vi "测试配置文件生成.vi"() -> ()   [LabVIEW 2013]
uses:
  <vilib>/Utility/config.llb/Write Key (String).vi
  <vilib>/Utility/config.llb/NI_LVConfig.lvlib
panel:
  in  "总电流":bool
  in  "外部总压":bool
  in  "内部总压":bool
  in  "选项卡控件":enum32{"关键配置", "功能测试"}(tab)
  in  "保存 2":bool
  in  "BMU合成程序全名-用于仿真器刷写":path
  in  "内部CAN波特率":enum16{"250K", "500K"}(ring)
  in  "整车CAN波特率":enum16{"250K", "500K"}(ring)
  in  "充电CAN波特率":enum16{"250K", "500K"}(ring)
  in  "BCU应用程序全名-用于在线更新程序":path
  in  "BMU个数":dbl
  in  "BMU应用程序全名 2":string[][](table)
  in  "BCU合成程序全名-用于仿真器刷写":path
  in  "配置文件全名":path
  in  "CP":bool
  in  "AI2":bool
  in  "AI1":bool
  in  "CC2":bool
  in  "CC":bool
  in  "全部忽略":bool
  in  "全部选择":bool
  in  "DO2":bool
  in  "DO1":bool
  in  "DI4":bool
  in  "DI3":bool
  in  "DI2":bool
  in  "DI1":bool
  in  "加热继电器":bool
  in  "风机继电器":bool
  in  "充电继电器":bool
  in  "预充继电器":bool
  in  "总负继电器":bool
  in  "总正继电器":bool
  in  "充电CAN":bool
  in  "整车CAN":bool
  in  "写入至从板号":dbl=1.0 min=1.0 max=30.0
  in  "更新至指定BMU号":bool
  in  "BMU应用程序全名":path
  in  "配置到全部BMU":bool
  out "取消":bool
  out "确定并启动":bool
  in  "自适就CAN卡类型":bool=TRUE
  in  "退出":bool
  in  "保存":bool
  in  "error in":errorcluster caption="错误输入"
  # "自动化测试配置文件生成器"
  # "将BMU应用程序全名："
  # "请勾选需要生产测试的功能........"
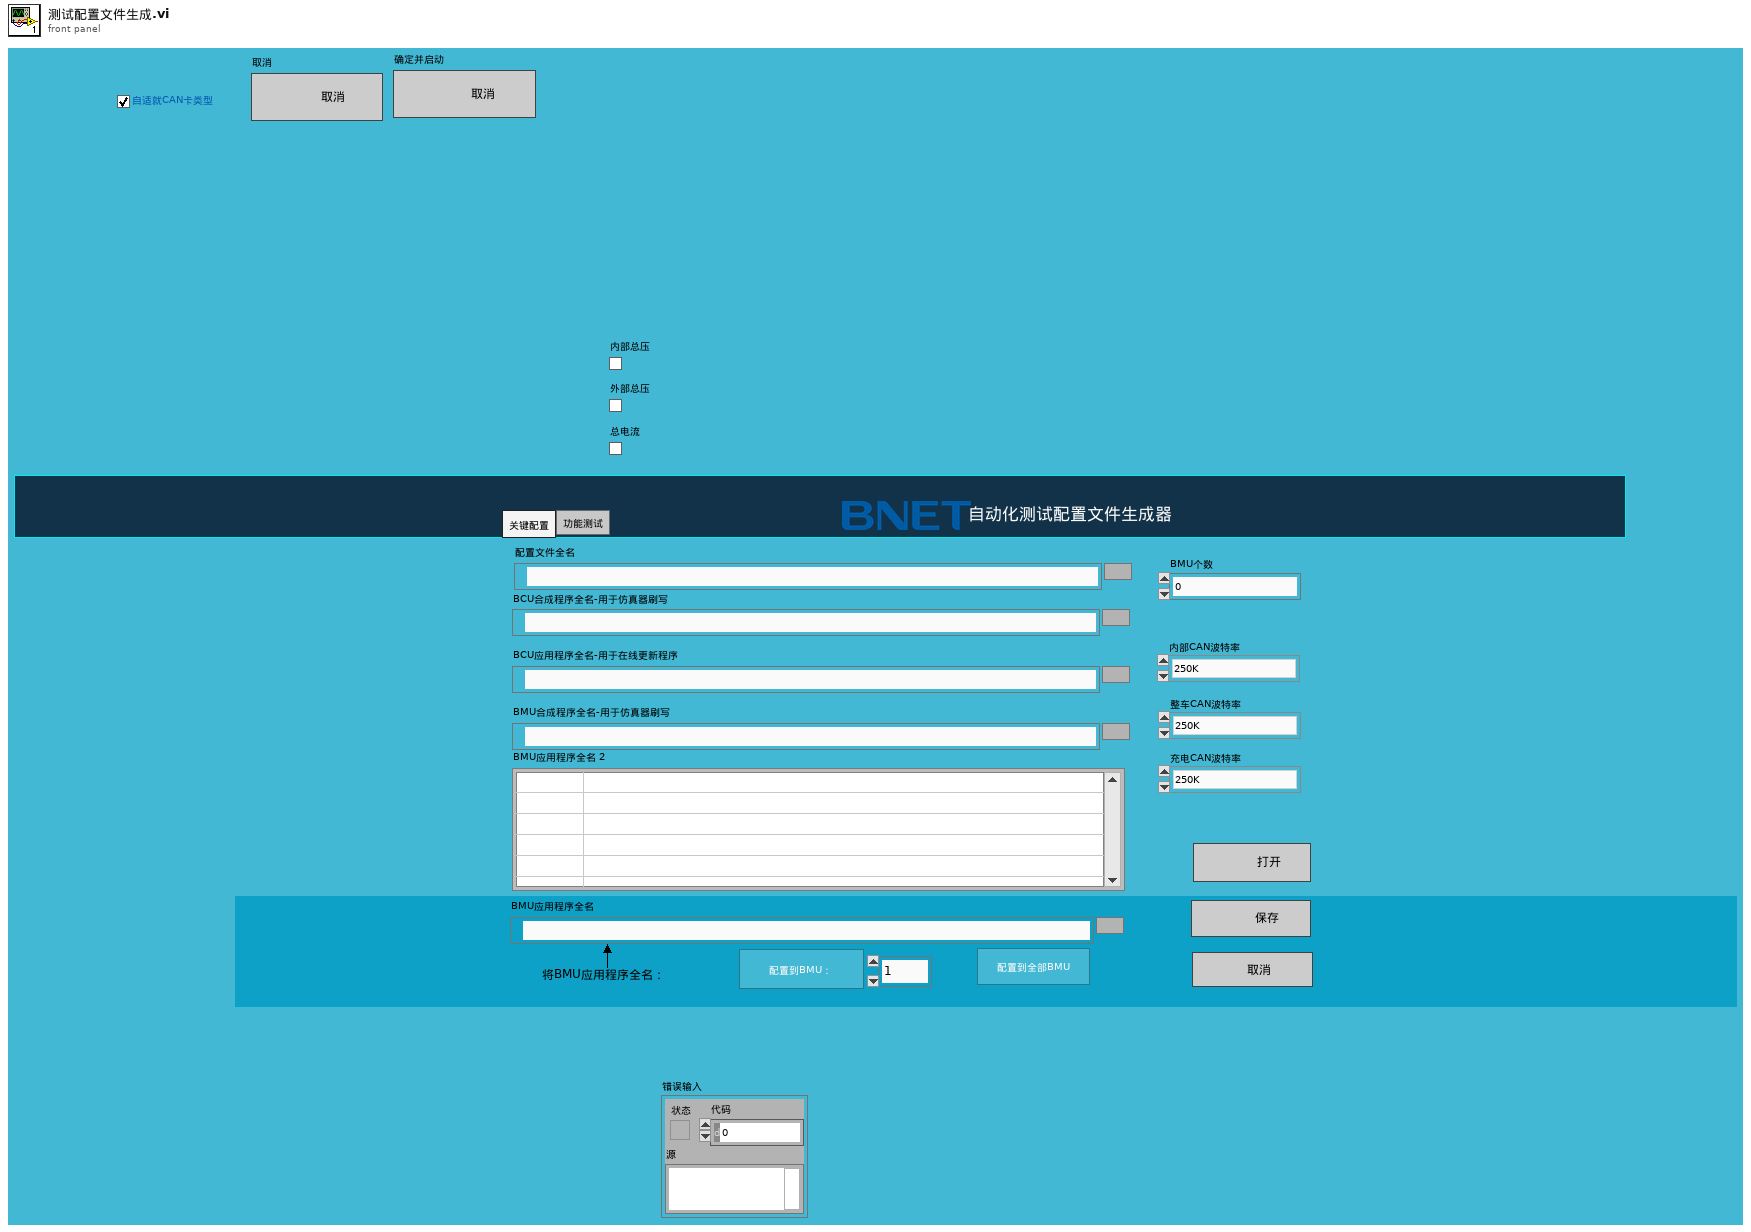
[diagram p1: front panel]
types:
  T1 = typedef "NI_LVConfig.lvlib/Config Data RefNum.ctl" = refnum<k1>
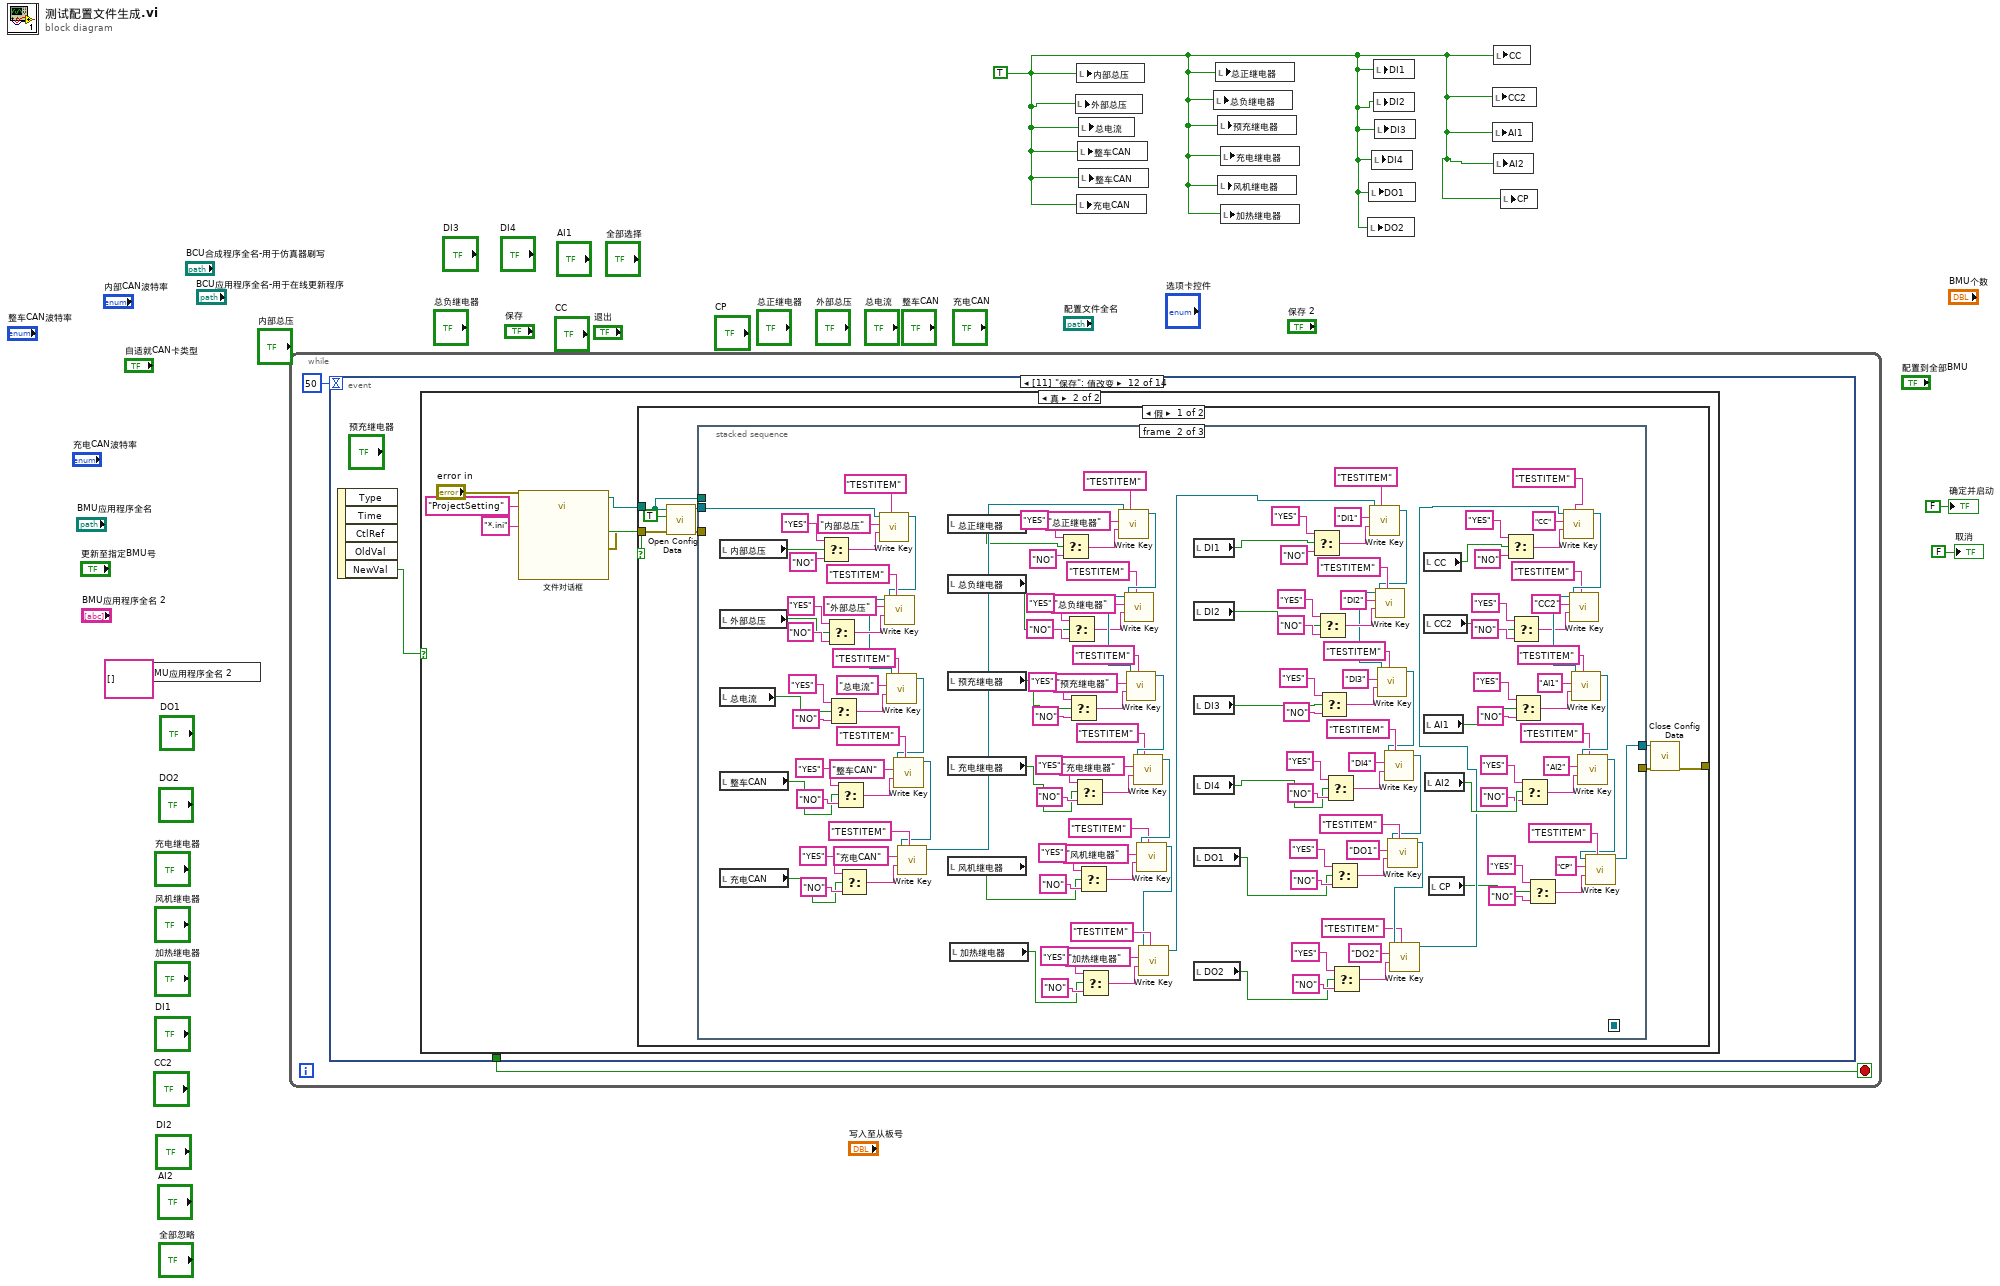
[diagram p0: block diagram]
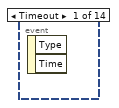
[diagram p2: hidden frame]
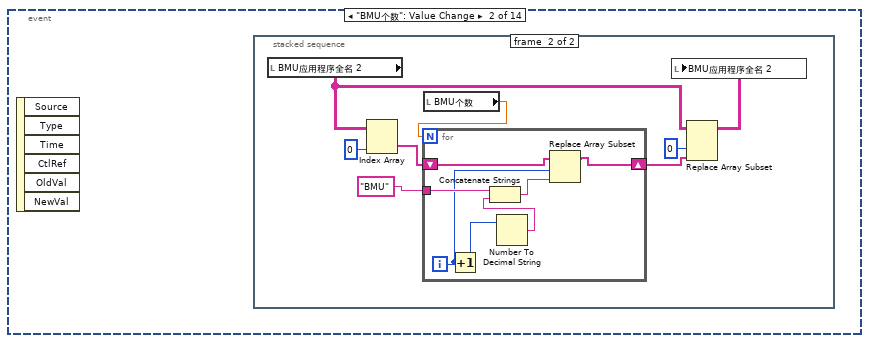
[diagram p3: hidden frame]
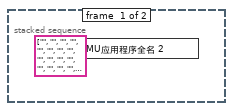
[diagram p4: hidden frame]
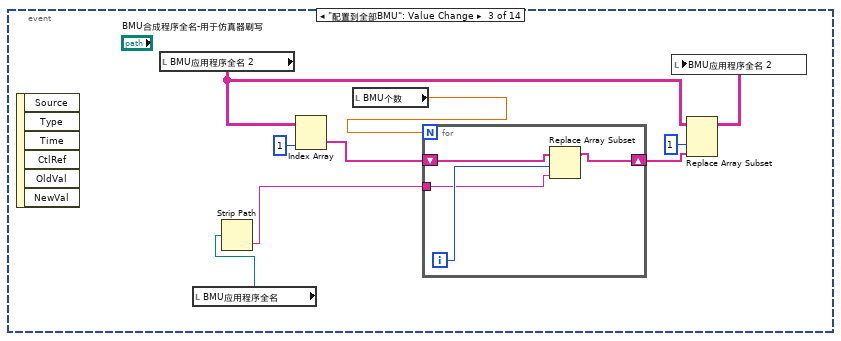
[diagram p5: hidden frame]
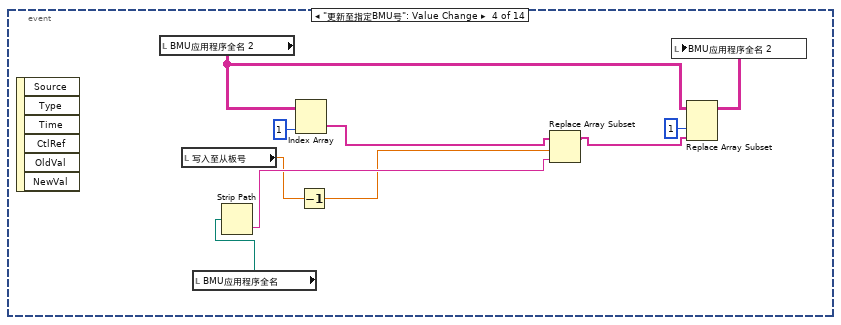
[diagram p6: hidden frame]
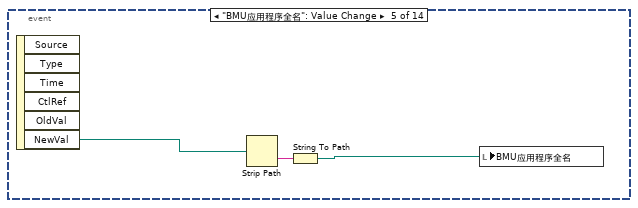
[diagram p7: hidden frame]
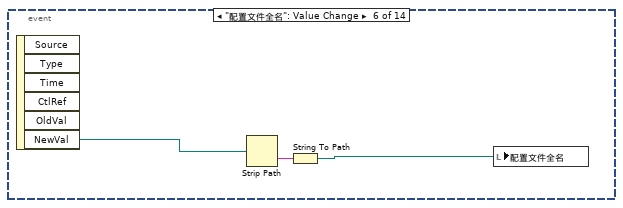
[diagram p8: hidden frame]
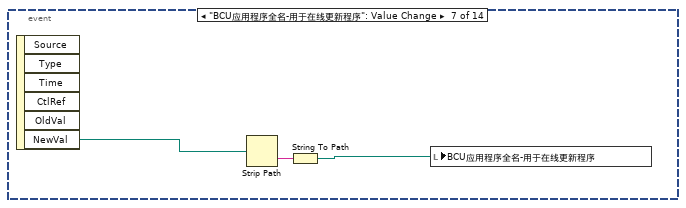
[diagram p9: hidden frame]
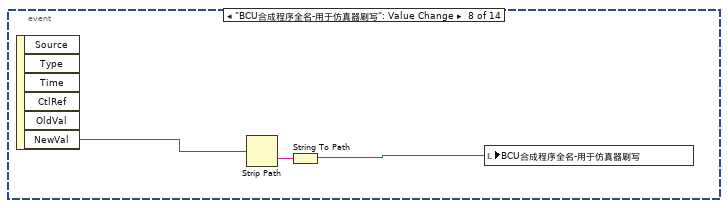
[diagram p10: hidden frame]
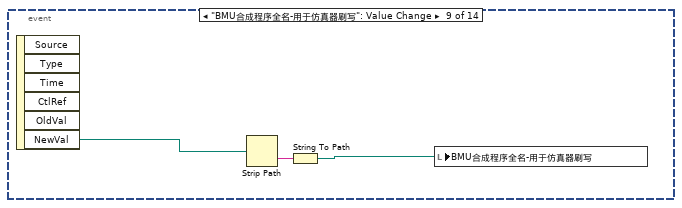
[diagram p11: hidden frame]
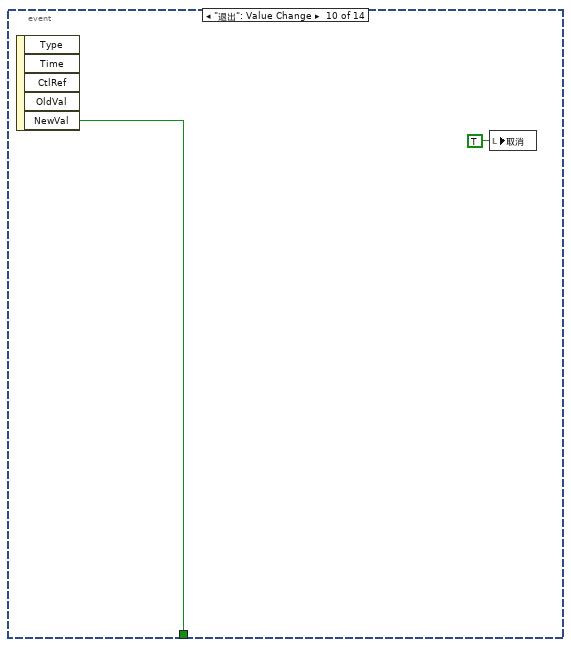
[diagram p12: hidden frame]
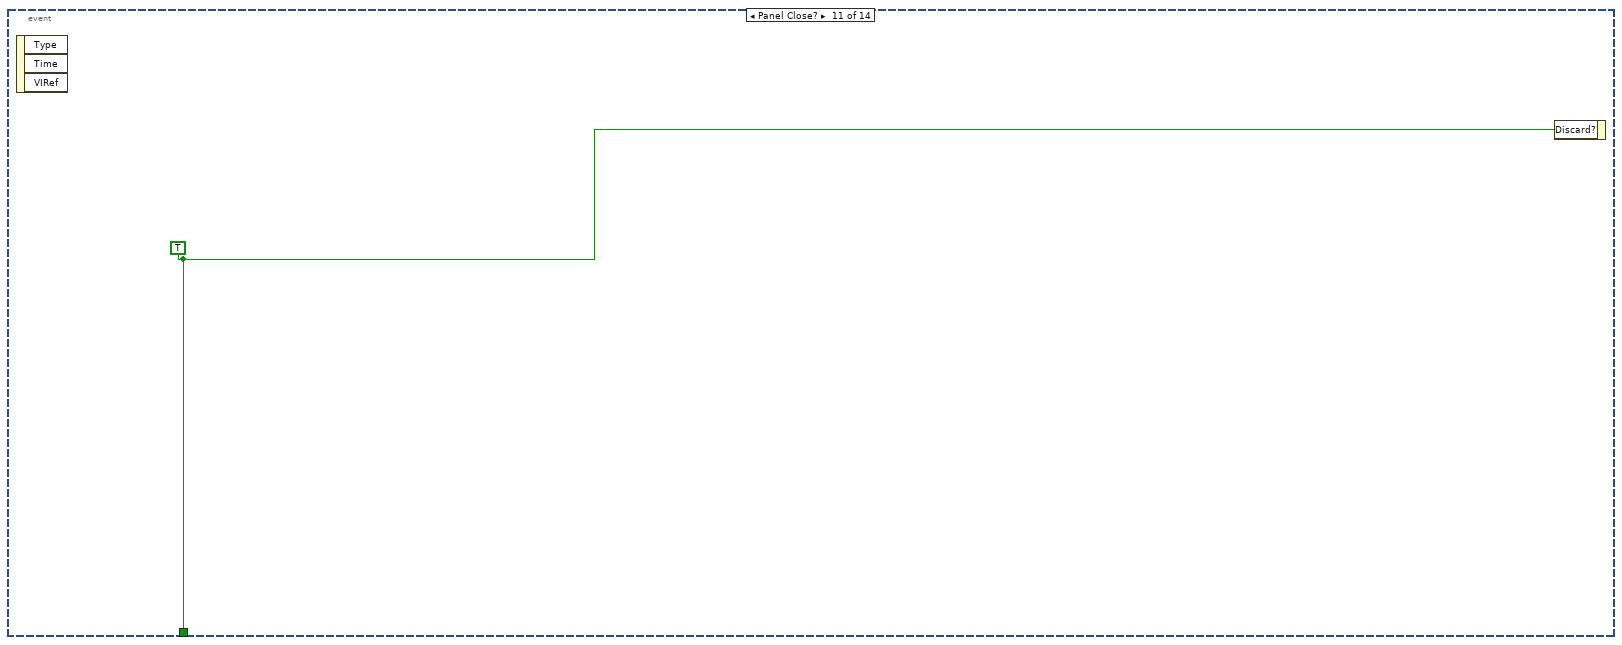
[diagram p13: hidden frame]
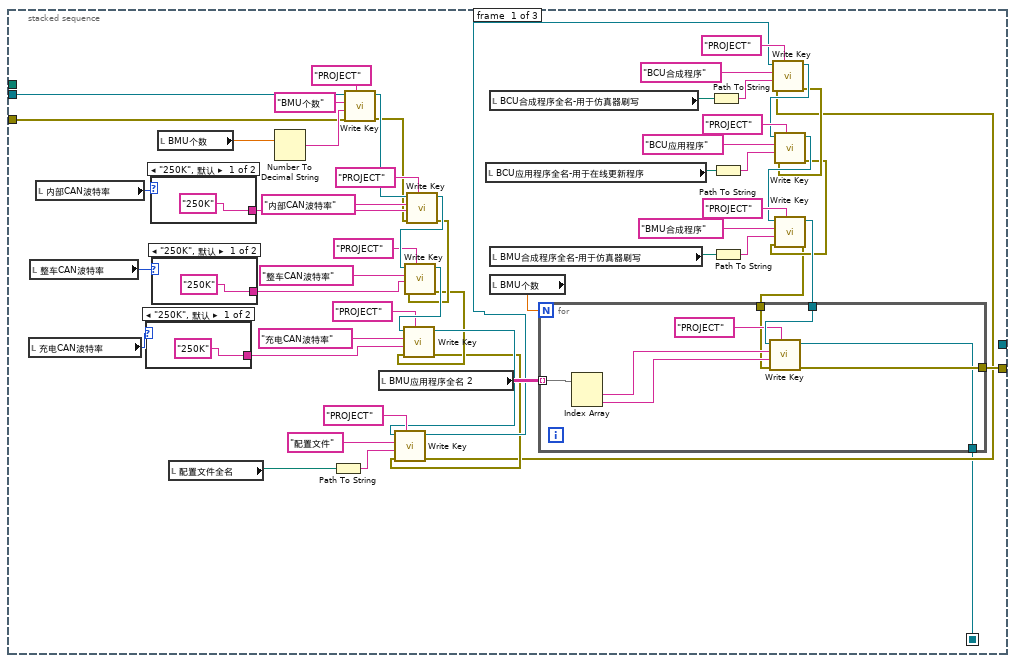
[diagram p15: hidden frame]
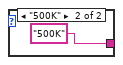
[diagram p16: hidden frame]
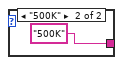
[diagram p17: hidden frame]
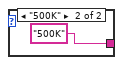
[diagram p18: hidden frame]
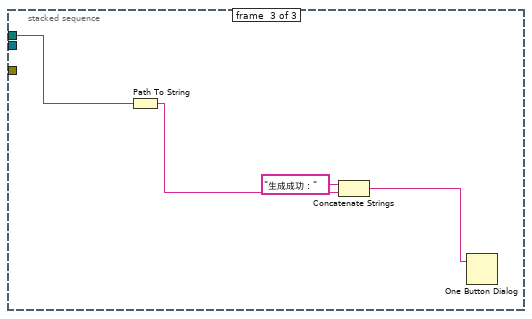
[diagram p19: hidden frame]
diagram:
  w1 = TRUE ("内部总压")
  n1 = local write "BMU应用程序全名 2"(string[][] [] ("从板路径")) -> ()
  n2 = while {
    stop <- w6 stop-if-true
    n3 = event shown="[11] \"保存\": 值改变" {
      selector: _ -> [_ _ _ _ _ _ _ _ _ _ _ _ _ _]
      dyn-events: _ -> [_ _ _ _ _ _ _ _ _ _ _ _ _ _]
      timeout: 50 -> [_ _ _ _ _ _ _ _ _ _ _ _ _ _]
      tunnel: [_ _ _ _ _ _ _ _ _ w62 w63 _ _ _] -> w6
      event Timeout {
        n4 = event-data() -> ()  [unwired: 3 out]
      }
      event "BMU个数": Value Change {
        n5 = event-data() -> ()  [unwired: 7 out]
        n6 = stacked-sequence {
          frame #0 {
            n7 = local write "BMU应用程序全名 2"(string[][] [["", "", ""], ["", "", ""], ["", "", ""], ["", "", ""], ["", "", ""], ["", "", ""], ["", "", ""], ["", "", ""], ["", "", ""], ["", "", ""], ["", "", ""], ["", "", ""], ["", "", ""], ["", "", ""], ["", "", ""], ["", "", ""], ["", "", ""], ["", "", ""], ["", "", ""], ["", "", ""], ["", "", ""], ["", "", ""], ["", "", ""], ["", "", ""], ["", "", ""], ["", "", ""], ["", "", ""], ["", "", ""], ["", "", ""], ["", "", ""], ["", "", " "]] ("从板路径")) -> ()
          }
          frame #1 {
            n8 = local read "BMU应用程序全名 2"() -> (w11:string[][])
            n9 = Index Array(array=w11, index (col)=0 ("禁用的索引 (列)")) -> (element=w14:string[])  [unwired: 1 in]
            n10 = local read "BMU个数"() -> (w13:dbl)
            n11 = for {
              N: w13 -> [_]
              tunnel: "BMU" -> [w20]
              shift-right: [w17] -> w9
              shift-left: w14 -> [w22]
              i -> [w16]
              n12 = Increment(x=w16) -> (x+1=w21:i32)
              n13 = Number To Decimal String(number=w21) -> (decimal integer string=w19:string)  [unwired: 1 in]
              n14 = Concatenate Strings(w20, w19) -> (w18:string)
              n15 = Replace Array Subset(array=w22, new element=w18, index=w16) -> (w17:string[])
            }
            n16 = Replace Array Subset(array=w11, new element=w9, index (col)=0 ("禁用的索引 (列)")) -> (w8:string[][])  [unwired: 1 in]
            n17 = local write "BMU应用程序全名 2"(w8) -> ()
          }
        }
      }
      event "配置到全部BMU": Value Change {
        n18 = event-data() -> ()  [unwired: 7 out]
        n19 = local read "BMU应用程序全名 2"() -> (w28:string[][])
        n20 = local read "BMU应用程序全名"() -> (w24:path)
        n21 = Strip Path(path=w24) -> (name=w23:string)  [unwired: 1 out]
        n22 = Index Array(array=w28, index (col)=1 ("禁用的索引 (列)")) -> (element=w30:string[])  [unwired: 1 in]
        n23 = local read "BMU个数"() -> (w29:dbl)
        n24 = for {
          N: w29 -> [_]
          tunnel: w23 -> [w32]
          shift-right: [w34] -> w26
          shift-left: w30 -> [w35]
          i -> [w33]
          n25 = Replace Array Subset(array=w35, new element=w32, index=w33) -> (w34:string[])
        }
        n26 = Replace Array Subset(array=w28, new element=w26, index (col)=1 ("禁用的索引 (列)")) -> (w25:string[][])  [unwired: 1 in]
        n27 = local write "BMU应用程序全名 2"(w25) -> ()
      }
      event "更新至指定BMU号": Value Change {
        n28 = event-data() -> ()  [unwired: 7 out]
        n29 = local read "BMU应用程序全名 2"() -> (w43:string[][])
        n30 = local read "写入至从板号"() -> (w37:dbl)
        n31 = local read "BMU应用程序全名"() -> (w39:path)
        n32 = Strip Path(path=w39) -> (name=w38:string)  [unwired: 1 out]
        n33 = Index Array(array=w43, index (col)=1 ("禁用的索引 (列)")) -> (element=w44:string[])  [unwired: 1 in]
        n34 = Decrement(x=w37) -> (x-1=w36:dbl)
        n35 = Replace Array Subset(array=w44, new element=w38, index=w36) -> (w41:string[])
        n36 = Replace Array Subset(array=w43, new element=w41, index (col)=1 ("禁用的索引 (列)")) -> (w40:string[][])  [unwired: 1 in]
        n37 = local write "BMU应用程序全名 2"(w40) -> ()
      }
      event "BMU应用程序全名": Value Change {
        n38 = event-data() -> ("NewVal"=w48:path)  [unwired: 6 out]
        n39 = Strip Path(path=w48) -> (name=w47:string)  [unwired: 1 out]
        n40 = String To Path(string=w47) -> (path=w46:path)
        n41 = local write "BMU应用程序全名"(w46) -> ()
      }
      event "配置文件全名": Value Change {
        n42 = event-data() -> ("NewVal"=w51:path)  [unwired: 6 out]
        n43 = Strip Path(path=w51) -> (name=w50:string)  [unwired: 1 out]
        n44 = String To Path(string=w50) -> (path=w49:path)
        n45 = local write "配置文件全名"(w49) -> ()
      }
      event "BCU应用程序全名-用于在线更新程序": Value Change {
        n46 = event-data() -> ("NewVal"=w54:path)  [unwired: 6 out]
        n47 = Strip Path(path=w54) -> (name=w53:string)  [unwired: 1 out]
        n48 = String To Path(string=w53) -> (path=w52:path)
        n49 = local write "BCU应用程序全名-用于在线更新程序"(w52) -> ()
      }
      event "BCU合成程序全名-用于仿真器刷写": Value Change {
        n50 = event-data() -> ("NewVal"=w57:path)  [unwired: 6 out]
        n51 = Strip Path(path=w57) -> (name=w56:string)  [unwired: 1 out]
        n52 = String To Path(string=w56) -> (path=w55:path)
        n53 = local write "BCU合成程序全名-用于仿真器刷写"(w55) -> ()
      }
      event "BMU合成程序全名-用于仿真器刷写": Value Change {
        n54 = event-data() -> ("NewVal"=w60:path)  [unwired: 6 out]
        n55 = Strip Path(path=w60) -> (name=w59:string)  [unwired: 1 out]
        n56 = String To Path(string=w59) -> (path=w58:path)
        n57 = local write "BMU合成程序全名-用于仿真器刷写"(w58) -> ()
      }
      event "退出": Value Change {
        n58 = event-data() -> ("NewVal"=w62:bool)  [unwired: 5 out]
        n59 = local write "取消"(TRUE ("取消")) -> ()
      }
      event Panel Close? {
        w63 = TRUE ("NewVal")
        n60 = event-data() -> ()  [unwired: 4 out]
        n61 = event-data("Discard?"=w63) -> ()  [unwired: 1 in, 1 out]
      }
      event "保存": Value Change {
        n62 = event-data() -> ("NewVal"=w64:bool)  [unwired: 5 out]
        n63 = case shown="真" w64 {
          frame False {
          }
          frame True {
            n64 = call "文件对话框"("default name"="ProjectSetting", "error in"="error in", "pattern (all files)"="*.ini") -> ("selected path"=w69:path, "cancelled"=w70:bool, "error out"=w65:errorcluster)  [unwired: 9 in, 1 out]
            n65 = case shown="假" w70 {
              tunnel: w69 -> [w71 _]
              tunnel: w65 -> [w75 _]
              tunnel: [w72 _] -> _
              frame False {
                n66 = call <vilib>:"Open Config Data.vi"("error in (no error)"=w75, "create file if necessary (T)"=TRUE, "configuration file path"=w71) -> ("error out"=w74:errorcluster, "refnum"=w77:T1)  [unwired: 6 in, 1 out]
                n67 = stacked-sequence {
                  seq-local: [w79 _ _] -> [_ _ _]
                  tunnel: w77 -> [w132 w155 _]
                  tunnel: [_ w148 _] -> w76
                  tunnel: w74 -> [w95 _ _]
                  tunnel: [w89 _ _] -> w73
                  tunnel: w71 -> [_ _ w305]
                  frame #0 {
                    n68 = local read "充电CAN波特率"() -> (w115:enum16{"250K", "500K"})
                    n69 = local read "整车CAN波特率"() -> (w118:enum16{"250K", "500K"})
                    n70 = local read "内部CAN波特率"() -> (w116:enum16{"250K", "500K"})
                    n71 = case shown="\"250K\", 默认" w115 {
                      tunnel: ["250K" ("key") "500K" ("key")] -> w97
                      frame "250K", Default {
                      }
                      frame "500K" {
                      }
                    }
                    n72 = case shown="\"250K\", 默认" w116 {
                      tunnel: ["250K" ("key") "500K" ("key")] -> w96
                      frame "250K", Default {
                      }
                      frame "500K" {
                      }
                    }
                    n73 = case shown="\"250K\", 默认" w118 {
                      tunnel: ["250K" ("key") "500K" ("key")] -> w117
                      frame "250K", Default {
                      }
                      frame "500K" {
                      }
                    }
                    n74 = local read "BMU个数"() -> (w129:dbl)
                    n75 = local read "配置文件全名"() -> (w87:path)
                    n76 = Number To Decimal String(number=w129) -> (decimal integer string=w128:string)  [unwired: 1 in]
                    n77 = Path To String(path=w87) -> (string=w88:string)
                    n78 = call-poly <vilib>:"Write Key.vi"("section"="PROJECT", "error in (no error)"=w95, "value"=w128, "key"="BMU个数", "refnum"=w132) -> ("error out"=w94:errorcluster, "refnum out"=w127:T1)  [unwired: 4 in, 1 out]
                    n79 = local read "BMU应用程序全名 2"() -> (w98:string[][])
                    n80 = call-poly <vilib>:"Write Key.vi"("section"="PROJECT", "error in (no error)"=w94, "value"=w96, "key"="内部CAN波特率", "refnum"=w127) -> ("error out"=w93:errorcluster, "refnum out"=w123:T1)  [unwired: 4 in, 1 out]
                    n81 = call-poly <vilib>:"Write Key.vi"("section"="PROJECT", "error in (no error)"=w93, "value"=w117, "key"="整车CAN波特率", "refnum"=w123) -> ("error out"=w82:errorcluster, "refnum out"=w122:T1)  [unwired: 4 in, 1 out]
                    n82 = call-poly <vilib>:"Write Key.vi"("section"="PROJECT", "error in (no error)"=w82, "value"=w97, "key"="充电CAN波特率", "refnum"=w122) -> ("error out"=w81:errorcluster, "refnum out"=w84:T1)  [unwired: 4 in, 1 out]
                    n83 = call-poly <vilib>:"Write Key.vi"("section"="PROJECT", "error in (no error)"=w81, "value"=w88, "key"="配置文件", "refnum"=w84) -> ("error out"=w80:errorcluster, "refnum out"=w83:T1)  [unwired: 4 in, 1 out]
                    n84 = local read "BCU应用程序全名-用于在线更新程序"() -> (w109:path)
                    n85 = local read "BCU合成程序全名-用于仿真器刷写"() -> (w112:path)
                    n86 = local read "BMU合成程序全名-用于仿真器刷写"() -> (w103:path)
                    n87 = local read "BMU个数"() -> (w99:dbl)
                    n88 = Path To String(path=w112) -> (string=w111:string)
                    n89 = Path To String(path=w109) -> (string=w110:string)
                    n90 = Path To String(path=w103) -> (string=w102:string)
                    n91 = call-poly <vilib>:"Write Key.vi"("section"="PROJECT", "error in (no error)"=w80, "value"=w111, "key"="BCU合成程序", "refnum"=w83) -> ("error out"=w92:errorcluster, "refnum out"=w106:T1)  [unwired: 4 in, 1 out]
                    n92 = call-poly <vilib>:"Write Key.vi"("section"="PROJECT", "error in (no error)"=w92, "value"=w110, "key"="BCU应用程序", "refnum"=w106) -> ("error out"=w91:errorcluster, "refnum out"=w101:T1)  [unwired: 4 in, 1 out]
                    n93 = call-poly <vilib>:"Write Key.vi"("section"="PROJECT", "error in (no error)"=w91, "value"=w102, "key"="BMU合成程序", "refnum"=w101) -> ("error out"=w90:errorcluster, "refnum out"=w100:T1)  [unwired: 4 in, 1 out]
                    n94 = for {
                      N: w99 -> [_]
                      tunnel: w100 -> [w140]
                      tunnel: w98 -> [w139] mode=indexing
                      tunnel: w90 -> [w135]
                      tunnel: [w134] -> w89
                      tunnel: [w133] -> w79
                      n95 = Index Array(array=w139) -> (element #1=w138:string, element #2=w137:string)  [unwired: 2 in]
                      n96 = call-poly <vilib>:"Write Key.vi"("section"="PROJECT", "error in (no error)"=w135, "value"=w137, "key"=w138, "refnum"=w140) -> ("error out"=w134:errorcluster, "refnum out"=w133:T1)  [unwired: 4 in, 1 out]
                    }
                  }
                  frame #1 {
                    n97 = local read "内部总压"() -> (w299:bool)
                    n98 = local read "外部总压"() -> (w271:bool)
                    n99 = local read "总电流"() -> (w270:bool)
                    n100 = local read "整车CAN"() -> (w269:bool)
                    n101 = local read "充电CAN"() -> (w268:bool)
                    n102 = Select(t="YES" ("key"), s=w299, f="NO" ("key")) -> (s? t:f=w296:string)
                    n103 = Select(t="YES" ("key"), s=w271, f="NO" ("key")) -> (s? t:f=w295:string)
                    n104 = Select(t="YES" ("key"), s=w270, f="NO" ("key")) -> (s? t:f=w286:string)
                    n105 = Select(t="YES" ("key"), s=w269, f="NO" ("key")) -> (s? t:f=w285:string)
                    n106 = Select(t="YES" ("key"), s=w268, f="NO" ("key")) -> (s? t:f=w276:string)
                    n107 = call-poly <vilib>:"Write Key.vi"("section"="TESTITEM", "value"=w296, "key"="内部总压", "refnum"=w155) -> ("refnum out"=w275:T1)  [unwired: 5 in, 2 out]
                    n108 = call-poly <vilib>:"Write Key.vi"("section"="TESTITEM", "value"=w295, "key"="外部总压", "refnum"=w275) -> ("refnum out"=w274:T1)  [unwired: 5 in, 2 out]
                    n109 = call-poly <vilib>:"Write Key.vi"("section"="TESTITEM", "value"=w286, "key"="总电流", "refnum"=w274) -> ("refnum out"=w273:T1)  [unwired: 5 in, 2 out]
                    n110 = call-poly <vilib>:"Write Key.vi"("section"="TESTITEM", "value"=w285, "key"="整车CAN", "refnum"=w273) -> ("refnum out"=w272:T1)  [unwired: 5 in, 2 out]
                    n111 = call-poly <vilib>:"Write Key.vi"("section"="TESTITEM", "value"=w276, "key"="充电CAN", "refnum"=w272) -> ("refnum out"=w233:T1)  [unwired: 5 in, 2 out]
                    n112 = local read "总正继电器"() -> (w232:bool)
                    n113 = local read "总负继电器"() -> (w231:bool)
                    n114 = local read "预充继电器"() -> (w230:bool)
                    n115 = local read "充电继电器"() -> (w229:bool)
                    n116 = local read "风机继电器"() -> (w228:bool)
                    n117 = local read "加热继电器"() -> (w227:bool)
                    n118 = Select(t="YES" ("key"), s=w232, f="NO" ("key")) -> (s? t:f=w243:string)
                    n119 = Select(t="YES" ("key"), s=w231, f="NO" ("key")) -> (s? t:f=w244:string)
                    n120 = Select(t="YES" ("key"), s=w230, f="NO" ("key")) -> (s? t:f=w253:string)
                    n121 = Select(t="YES" ("key"), s=w229, f="NO" ("key")) -> (s? t:f=w254:string)
                    n122 = Select(t="YES" ("key"), s=w228, f="NO" ("key")) -> (s? t:f=w263:string)
                    n123 = Select(t="YES" ("key"), s=w227, f="NO" ("key")) -> (s? t:f=w234:string)
                    n124 = call-poly <vilib>:"Write Key.vi"("section"="TESTITEM", "value"=w243, "key"="总正继电器", "refnum"=w233) -> ("refnum out"=w264:T1)  [unwired: 5 in, 2 out]
                    n125 = call-poly <vilib>:"Write Key.vi"("section"="TESTITEM", "value"=w244, "key"="总负继电器", "refnum"=w264) -> ("refnum out"=w265:T1)  [unwired: 5 in, 2 out]
                    n126 = call-poly <vilib>:"Write Key.vi"("section"="TESTITEM", "value"=w253, "key"="预充继电器", "refnum"=w265) -> ("refnum out"=w266:T1)  [unwired: 5 in, 2 out]
                    n127 = call-poly <vilib>:"Write Key.vi"("section"="TESTITEM", "value"=w254, "key"="充电继电器", "refnum"=w266) -> ("refnum out"=w267:T1)  [unwired: 5 in, 2 out]
                    n128 = call-poly <vilib>:"Write Key.vi"("section"="TESTITEM", "value"=w263, "key"="风机继电器", "refnum"=w267) -> ("refnum out"=w226:T1)  [unwired: 5 in, 2 out]
                    n129 = call-poly <vilib>:"Write Key.vi"("section"="TESTITEM", "value"=w234, "key"="加热继电器", "refnum"=w226) -> ("refnum out"=w184:T1)  [unwired: 5 in, 2 out]
                    n130 = local read "DI1"() -> (w190:bool)
                    n131 = local read "DI2"() -> (w189:bool)
                    n132 = local read "DI3"() -> (w188:bool)
                    n133 = local read "DI4"() -> (w187:bool)
                    n134 = local read "DO1"() -> (w186:bool)
                    n135 = local read "DO2"() -> (w185:bool)
                    n136 = Select(t="YES" ("key"), s=w190, f="NO" ("key")) -> (s? t:f=w215:string)
                    n137 = Select(t="YES" ("key"), s=w189, f="NO" ("key")) -> (s? t:f=w214:string)
                    n138 = Select(t="YES" ("key"), s=w188, f="NO" ("key")) -> (s? t:f=w205:string)
                    n139 = Select(t="YES" ("key"), s=w187, f="NO" ("key")) -> (s? t:f=w204:string)
                    n140 = Select(t="YES" ("key"), s=w186, f="NO" ("key")) -> (s? t:f=w195:string)
                    n141 = Select(t="YES" ("key"), s=w185, f="NO" ("key")) -> (s? t:f=w224:string)
                    n142 = call-poly <vilib>:"Write Key.vi"("section"="TESTITEM", "value"=w215, "key"="DI1", "refnum"=w184) -> ("refnum out"=w194:T1)  [unwired: 5 in, 2 out]
                    n143 = call-poly <vilib>:"Write Key.vi"("section"="TESTITEM", "value"=w214, "key"="DI2", "refnum"=w194) -> ("refnum out"=w193:T1)  [unwired: 5 in, 2 out]
                    n144 = call-poly <vilib>:"Write Key.vi"("section"="TESTITEM", "value"=w205, "key"="DI3", "refnum"=w193) -> ("refnum out"=w192:T1)  [unwired: 5 in, 2 out]
                    n145 = call-poly <vilib>:"Write Key.vi"("section"="TESTITEM", "value"=w204, "key"="DI4", "refnum"=w192) -> ("refnum out"=w191:T1)  [unwired: 5 in, 2 out]
                    n146 = call-poly <vilib>:"Write Key.vi"("section"="TESTITEM", "value"=w195, "key"="DO1", "refnum"=w191) -> ("refnum out"=w225:T1)  [unwired: 5 in, 2 out]
                    n147 = call-poly <vilib>:"Write Key.vi"("section"="TESTITEM", "value"=w224, "key"="DO2", "refnum"=w225) -> ("refnum out"=w157:T1)  [unwired: 5 in, 2 out]
                    n148 = local read "CC"() -> (w162:bool)
                    n149 = local read "CC2"() -> (w161:bool)
                    n150 = local read "AI1"() -> (w160:bool)
                    n151 = local read "AI2"() -> (w159:bool)
                    n152 = local read "CP"() -> (w147:bool)
                    n153 = Select(t="YES" ("key"), s=w162, f="NO" ("key")) -> (s? t:f=w166:string)
                    n154 = Select(t="YES" ("key"), s=w161, f="NO" ("key")) -> (s? t:f=w167:string)
                    n155 = Select(t="YES" ("key"), s=w160, f="NO" ("key")) -> (s? t:f=w176:string)
                    n156 = Select(t="YES" ("key"), s=w159, f="NO" ("key")) -> (s? t:f=w177:string)
                    n157 = Select(t="YES" ("key"), s=w147, f="NO" ("key")) -> (s? t:f=w153:string)
                    n158 = call-poly <vilib>:"Write Key.vi"("section"="TESTITEM", "value"=w166, "key"="CC", "refnum"=w157) -> ("refnum out"=w181:T1)  [unwired: 5 in, 2 out]
                    n159 = call-poly <vilib>:"Write Key.vi"("section"="TESTITEM", "value"=w167, "key"="CC2", "refnum"=w181) -> ("refnum out"=w182:T1)  [unwired: 5 in, 2 out]
                    n160 = call-poly <vilib>:"Write Key.vi"("section"="TESTITEM", "value"=w176, "key"="AI1", "refnum"=w182) -> ("refnum out"=w183:T1)  [unwired: 5 in, 2 out]
                    n161 = call-poly <vilib>:"Write Key.vi"("section"="TESTITEM", "value"=w177, "key"="AI2", "refnum"=w183) -> ("refnum out"=w149:T1)  [unwired: 5 in, 2 out]
                    n162 = call-poly <vilib>:"Write Key.vi"("section"="TESTITEM", "value"=w153, "key"="CP", "refnum"=w149) -> ("refnum out"=w148:T1)  [unwired: 5 in, 2 out]
                  }
                  frame #2 {
                    n163 = Path To String(path=w305) -> (string=w304:string)
                    n164 = Concatenate Strings("生成成功：" ("字符串"), w304) -> (w302:string)
                    n165 = One Button Dialog(message=w302) -> ()  [unwired: 1 in, 1 out]
                  }
                }
                n166 = call <vilib>:"Close Config Data.vi"("error in (no error)"=w73, "refnum"=w76) -> ("error out"=w72:errorcluster)  [unwired: 8 in, 1 out]
              }
              frame True {
              }
            }
          }
        }
      }
      event "全部选择": Value Change {
        n167 = event-data() -> ("NewVal"=w306:bool)  [unwired: 6 out]
        n168 = case shown="真" w306 {
          frame False {
          }
          frame True {
            w307 = TRUE ("内部总压")
            n169 = local write "外部总压"(w307) -> ()
            n170 = local write "内部总压"(w307) -> ()
            n171 = local write "充电CAN"(w307) -> ()
            n172 = local write "整车CAN"(w307) -> ()
            n173 = local write "总电流"(w307) -> ()
            n174 = local write "整车CAN"(w307) -> ()
            n175 = local write "总负继电器"(w307) -> ()
            n176 = local write "总正继电器"(w307) -> ()
            n177 = local write "预充继电器"(w307) -> ()
            n178 = local write "风机继电器"(w307) -> ()
            n179 = local write "充电继电器"(w307) -> ()
            n180 = local write "加热继电器"(w307) -> ()
            n181 = local write "DO2"(w307) -> ()
            n182 = local write "DO1"(w307) -> ()
            n183 = local write "DI4"(w307) -> ()
            n184 = local write "DI1"(w307) -> ()
            n185 = local write "DI2"(w307) -> ()
            n186 = local write "DI3"(w307) -> ()
            n187 = local write "CP"(w307) -> ()
            n188 = local write "CC2"(w307) -> ()
            n189 = local write "AI1"(w307) -> ()
            n190 = local write "CC"(w307) -> ()
            n191 = local write "AI2"(w307) -> ()
          }
        }
      }
      event "全部忽略": Value Change {
        n192 = event-data() -> ("NewVal"=w308:bool)  [unwired: 6 out]
        n193 = case shown="真" w308 {
          frame False {
          }
          frame True {
            w309 = FALSE ("内部总压")
            n194 = local write "外部总压"(w309) -> ()
            n195 = local write "内部总压"(w309) -> ()
            n196 = local write "充电CAN"(w309) -> ()
            n197 = local write "整车CAN"(w309) -> ()
            n198 = local write "总电流"(w309) -> ()
            n199 = local write "整车CAN"(w309) -> ()
            n200 = local write "总负继电器"(w309) -> ()
            n201 = local write "总正继电器"(w309) -> ()
            n202 = local write "预充继电器"(w309) -> ()
            n203 = local write "风机继电器"(w309) -> ()
            n204 = local write "充电继电器"(w309) -> ()
            n205 = local write "加热继电器"(w309) -> ()
            n206 = local write "DO2"(w309) -> ()
            n207 = local write "DO1"(w309) -> ()
            n208 = local write "DI4"(w309) -> ()
            n209 = local write "DI1"(w309) -> ()
            n210 = local write "DI2"(w309) -> ()
            n211 = local write "DI3"(w309) -> ()
            n212 = local write "CC2"(w309) -> ()
            n213 = local write "AI1"(w309) -> ()
            n214 = local write "CC"(w309) -> ()
            n215 = local write "AI2"(w309) -> ()
            n216 = local write "CP"(w309) -> ()
          }
        }
      }
    }
  }
  n217 = local write "外部总压"(w1) -> ()
  n218 = local write "内部总压"(w1) -> ()
  n219 = local write "充电CAN"(w1) -> ()
  n220 = local write "整车CAN"(w1) -> ()
  n221 = local write "总电流"(w1) -> ()
  n222 = local write "整车CAN"(w1) -> ()
  n223 = local write "总负继电器"(w1) -> ()
  n224 = local write "总正继电器"(w1) -> ()
  n225 = local write "预充继电器"(w1) -> ()
  n226 = local write "风机继电器"(w1) -> ()
  n227 = local write "充电继电器"(w1) -> ()
  n228 = local write "加热继电器"(w1) -> ()
  n229 = local write "DO2"(w1) -> ()
  n230 = local write "DO1"(w1) -> ()
  n231 = local write "DI4"(w1) -> ()
  n232 = local write "DI1"(w1) -> ()
  n233 = local write "DI2"(w1) -> ()
  n234 = local write "DI3"(w1) -> ()
  n235 = local write "CC2"(w1) -> ()
  n236 = local write "AI1"(w1) -> ()
  n237 = local write "CC"(w1) -> ()
  n238 = local write "AI2"(w1) -> ()
  n239 = local write "CP"(w1) -> ()
  "确定并启动" <- FALSE ("确定并启动")
  "取消" <- FALSE ("取消")
